vi "GUI for Real Encoder Test.vi"() -> ()   [LabVIEW 2009]
uses:
  <vilib>/userDefined/High Color/nirio_resource_hc.ctl
  <vilib>/rvi/interface/nirviOpenFPGA/nirviOpenFPGA.xnode
  FPGA Bitfiles/Athena Brain.lvproj_FPGA Target 2_RealEncoderTest.vi.lvbitx
  <vilib>/FPGAPlugInAG/sbRIO-9642/nirviIntfOpen_sbRIO-9642.vi
  <vilib>/rvi/interface/nirviReadWriteControl/nirviReadWriteControl.xnode
  <vilib>/Utility/error.llb/Error Cluster From Error Code.vi
  <vilib>/rvi/errors/niLvFpgaAdjustHostInterfaceError.vi
  <vilib>/rvi/interface/common/niFpgaNodeNameForErrorReporting.ctl
  <vilib>/rvi/errors/niLvFpgaWhatHappensToTopLevelVI.ctl
  NiRioSrv.dll
panel:
  in  "resource name":T1
  out "The Steering Encoder Changed":bool
  out "Current Steering Encoder Value":i32
  out "Maximum Steering Encoder Count":i32
  out "Minimum Steering Encoder Count":i32
  out "The Lidar Encoder Changed":bool
  out "Current Lidar Encoder Value":i32
  out "Maximum Lidar Encoder Count":i32
  out "Minimum Lidar Encoder Count":i32
  out "Minimum Drive Encoder Count":i32
  out "Maximum Drive Encoder Count":i32
  out "Current Drive Encoder Value":i32
  out "The Drive Encoder Changed":bool
  out "Steering Encoder A":bool
  out "Steering Encoder B":bool
  out "Steering Encoder Index":bool
  out "Lidar Encoder A":bool
  out "Lidar Encoder B":bool
  out "Lidar Encoder Index":bool
  out "Drive Encoder A":bool
  out "Drive Encoder B":bool
  out "Drive Encoder Index":bool
  in  "stop":bool
  in  "Lidar Enable":bool
  in  "Steering Enable":bool
  in  "Drive Enable":bool
  in  "Lidar output Voltage":fxp<+/-,20,5>
  in  "Steering output Voltage":fxp<+/-,20,5>
  in  "Drive output Voltage":fxp<+/-,20,5>
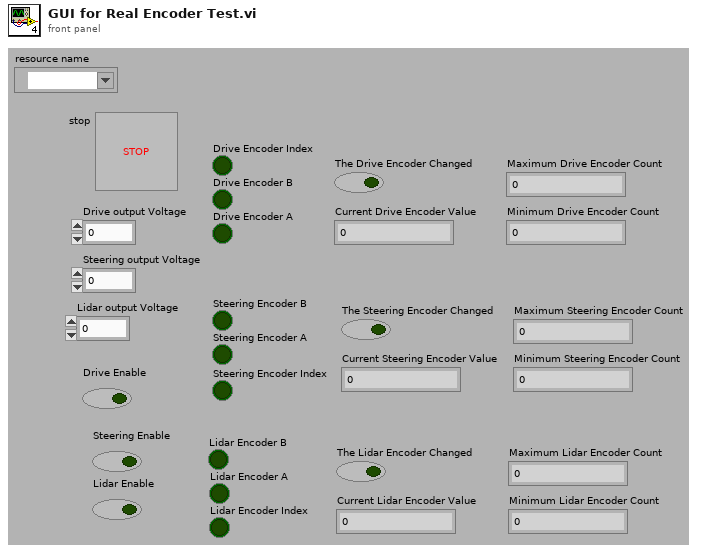
[diagram p1: front panel]
types:
  T1 = typedef "nirio_resource_hc.ctl" = tag
  T2 = typedef "niFpgaNodeNameForErrorReporting.ctl" = enum16{"Open FPGA VI Reference", "Read/Write Control", "Invoke Method: Abort", "Invoke Method: Acknowledge IRQ", "Invoke Method: Download", "Invoke Method: FIFO.Configure", "Invoke Method: FIFO.Read", "Invoke Method: FIFO.Start", "Invoke Method: FIFO.Stop", "Invoke Method: FIFO.Write", "Invoke Method: Reset", "Invoke Method: Run", "Invoke Method: Wait on IRQ", "Close FPGA VI Reference"}
  T3 = typedef "niLvFpgaWhatHappensToTopLevelVI.ctl" = enum16{"top level VI scripted behind XNode", "top level VI inlined behind XNode"}
  T4 = cluster{"signature":u8[], "vi signatures match":bool, "signature register address":u32, "reset register address":u32, "control register address":u32, "interrupt base address":u32, "Bitstream Version":u32, "DMA Configuration":cluster{"Name":string, "Depth":u32, "Write? (Deprecated:Use Implementation)":bool, "Physical Channel":u32, "Base Address":u32, "Data Width":u32, "Data Type":enum32{"Boolean", "I8", "I16", "I32", "I64", "U8", "U16", "U32", "U64", "FXP"}, "FXP Properties":variant, "Write Window Address":u32, "Implementation":enum16{"niFpgaTargetToHost", "niFpgaHostToTarget", "niFpgaPeerToPeerWriter", "niFpgaPeerToPeerReader", "niCoreTargetToHost", "niCoreHostToTarget"}, "Control Set":u32}[], "run when loaded?":bool, "reset register size in bits":u32, "compilation results xml":string}
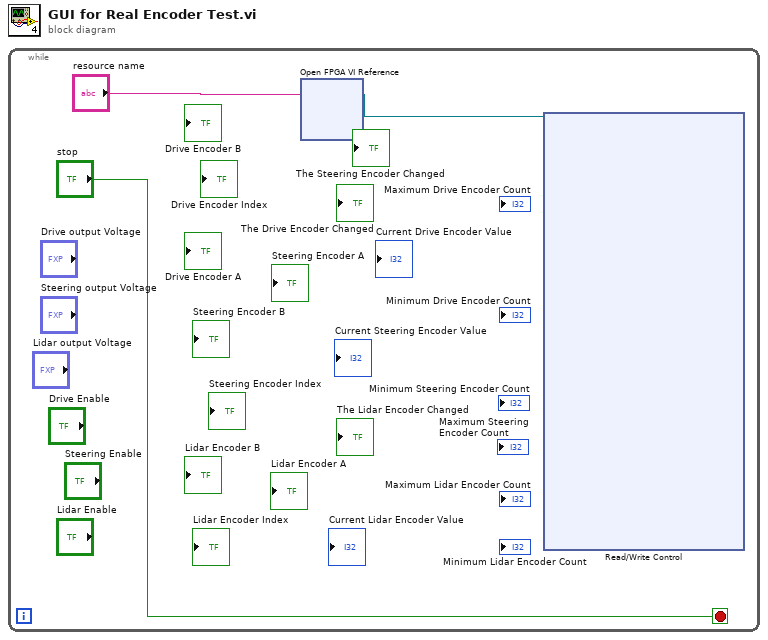
[diagram p0: block diagram]
diagram:
  n1 = while {
    stop <- "stop" stop-if-true
    n2 = xnode "Open FPGA VI Reference"("resource name"="resource name") -> ("FPGA VI Reference Out"=w2:refnum<k20>)  [unwired: 1 in, 1 out]
    n3 = xnode "Read/Write Control"("FPGA VI Reference In"=w2) -> ()  [unwired: 8 in, 23 out]
  }
